vi "Line Detector Fit Lorentzian.vi"(6 "Guess":dbl[](array[numeric]), 7 "Frequency":dbl[](array[numeric]), 8 "Error In":errorcluster, 10 "Signal":cdb[](array[numeric]), 11 "Line Detector Configuration":T1={"Peak width guess"=100.0, "Background removal"=enum."NONE", "Smoothing"=enum."NONE", "Smooth window"=100.0, "Relative threshold"=0.0, "Finder algorithm"=enum."Basic", "Bgd window"=100.0, "Spectrum recorder module name"="Spectrum Recorder", "Fit window"=100.0, "Initial fit guess"=enum."Peak finder", "Follow\npeaks"=FALSE, "Re-sample"=nan} {"Re-sample" format="%#_6pHz"; "Fit window" format="%#_6pHz"; "Bgd window" format="%#_6pHz"; "Smooth window" format="%#_6pHz"; "Peak width guess" format="%#_6pHz"}) -> (0 "Error Out":errorcluster, 1 "good fit?":dbl, 2 "Plot":cluster{"X":dbl[], "Array":dbl[]}[](array[cluster]), 3 "best fit parameters":dbl[](array[numeric]))   [LabVIEW 2016]
uses:
  LabActor/Post-Processors/Line Detector/Resonance Detector Configuration.ctl
panel:
  # "F0\n\nAmpl\n\nWidth"
  # "Peak finder config"
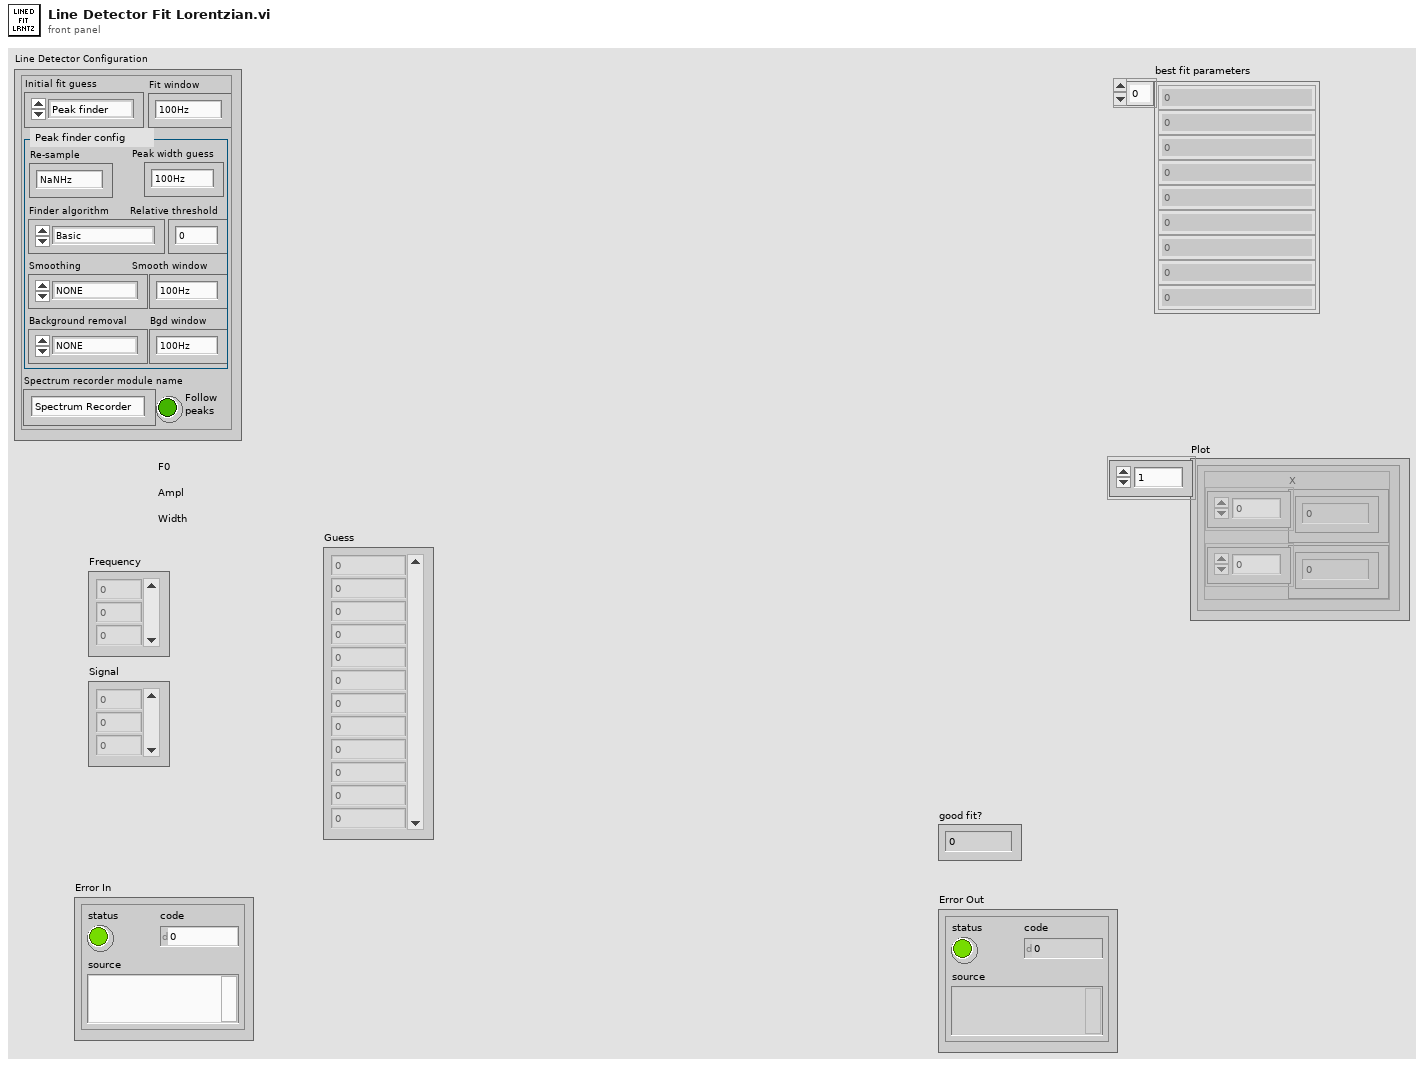
[diagram p1: front panel]
types:
  T1 = typedef "Resonance Detector Configuration.ctl" = cluster{"Peak width guess":dbl, "Background removal":enum16{"NONE", "High-pass", "Detrend"}, "Smoothing":enum16{"NONE", "Low-pass", "Denoise"}, "Smooth window":dbl, "Relative threshold":dbl, "Finder algorithm":enum16{"Basic", "Wavelet", "Wavelet+detrend"}, "Bgd window":dbl, "Spectrum recorder module name":string, "Fit window":dbl, "Initial fit guess":enum16{"Peak finder", "Last fit"}, "Follow\npeaks":bool, "Re-sample":dbl}
  T2 = cluster{"parameter minimum":dbl[], "parameter maximum":dbl[]}
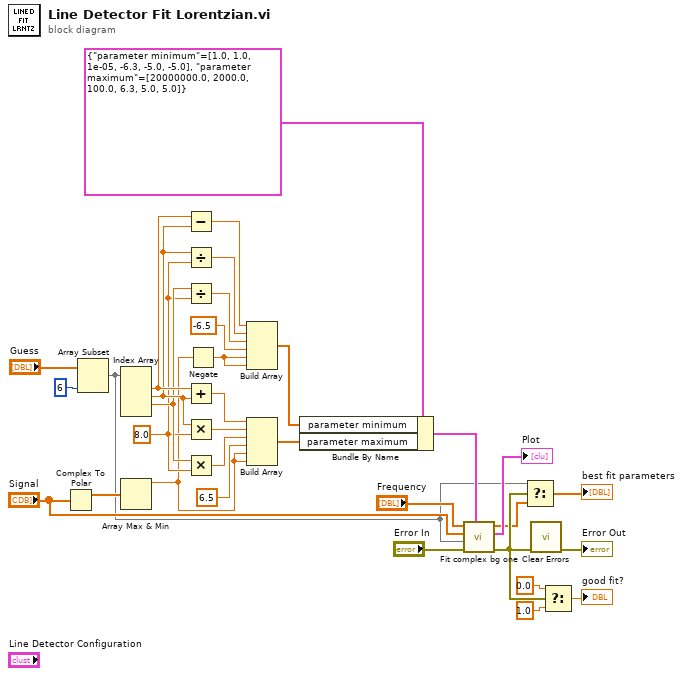
[diagram p0: block diagram]
diagram:
  w16 = 8.0
  n1 = Complex To Polar(r * e^(i*theta)="Signal") -> (r=w12:dbl[])  [unwired: 1 out]
  n2 = Array Subset(array="Guess", length=6) -> (w1:dbl[])  [unwired: 1 in]
  n3 = Index Array(array=w1) -> (element #1=w28:dbl, element #2=w26:dbl, element #3=w18:dbl)  [unwired: 4 in, 1 out]
  n4 = Array Max & Min(array=w12) -> (max value=w11:dbl)  [unwired: 3 out]
  n5 = Subtract(x=w28, y=w26) -> (x-y=w29:dbl)
  n6 = Divide(x=w26, y=w16) -> (x/y=w15:dbl)
  n7 = Divide(x=w18, y=w16) -> (x/y=w19:dbl)
  n8 = Add(x=w28, y=w26) -> (x+y=w27:dbl)
  n9 = Multiply(x=w26, y=w16) -> (x*y=w25:dbl)
  n10 = Multiply(x=w18, y=w16) -> (x*y=w17:dbl)
  n11 = Negate(x=w11) -> (-x=w22:dbl)
  n12 = Build Array(w29, w15, w19, -6.5 ("element"), w22, w22) -> (w24:dbl[])
  n13 = Build Array(w27, w25, w17, 6.5 ("element"), w11, w11) -> (w23:dbl[])
  n14 = Bundle By Name(cluster=T2 {"parameter minimum"=[1.0, 1.0, 1e-05, -6.3, -5.0, -5.0], "parameter maximum"=[20000000.0, 2000.0, 100.0, 6.3, 5.0, 5.0]} ("Bounds"), "parameter minimum"=w24, "parameter maximum"=w23) -> (w30:T2)
  n15 = call "Fit complex bg one.vi"("Bounds"=w30, "Error In"="Error In", "Initial parameters"=w1, "Z"="Signal", "X"="Frequency") -> ("Error Out"=w4:errorcluster, "Plot"=→"Plot":cluster{"X":dbl[], "Array":dbl[]}[], "best fit parameters"=w3:dbl[])  [unwired: 4 in]
  n16 = Select(t=w1, s=w4, f=w3) -> (s? t:f=→"best fit parameters":dbl[])
  n17 = call <vilib>:"Clear Errors.vi"("error in (no error)"=w4) -> ("error out"=→"Error Out":errorcluster)  [unwired: 5 in, 1 out]
  n18 = Select(t=0.0, s=w4, f=1.0 ("t")) -> (s? t:f=→"good fit?":dbl)
